vi "Write TaskConfig.vi"(8 "error in (no error)":errorcluster, 10 "TaskConfig":T1={"Drive"=enum."NI_DAQmx", "TaskType"=enum."AI", "PhysicalChannels"="", "SampleRateConfiguration"={"SampleRate"=0.0, "SamplesPerChannel"=0, "SamplesPerRead"=0, "SampleMode"=10123, "Clock Source"="OnboardClock"}, "ChannelConfig"={}, "Enable"=FALSE, "Original"=FALSE} {"SampleRateConfiguration"."SampleMode" items=["Finite Samples"=10178, "Continuous Samples"=10123, "Hardware Timed Single Point"=12522]}, 11 "Angular_Task in":refnum<class "Angular_Task.lvclass">) -> (0 "error out":errorcluster, 3 "Angular_Task out":refnum<class "Angular_Task.lvclass">)   [LabVIEW 2025, in "Angular_Task.lvlib" / "Angular_Task.lvclass"]
uses:
  Angular_Task.lvclass
  DAQ_Module/DAQ_Module/DAQ_Module/DAQ_Task_Config.ctl
  DAQ_Module/DAQ_Module/DAQ_Module/DAQ_HW_Type.ctl
  DAQ_Module/DAQ_Module/DAQ_Module/DAQ_Task_Type.ctl
  DAQ_Module/DAQ_Module/DAQ_Module/DAQ_SampleRateConfig.ctl
  DAQ_Module/DAQ_Module/DAQ_Module/DAQ_Angular_Task_Config.ctl
  e3aac5b7-c646-4fcd-a3ef-a0d2258a22a5.vi
  <vilib>/JDP Science/JSONtext/JSON text to Variant.vi
  Waveform_Task/Waveform_Task/Waveform_Task.lvclass
  <vilib>/JDP Science/JSONtext/LVClass Serializer/JSONtext LVClass Serializer.lvclass
  DAQ_Module/DAQ_Module/DAQ_Module/DAQ_Module.lvclass
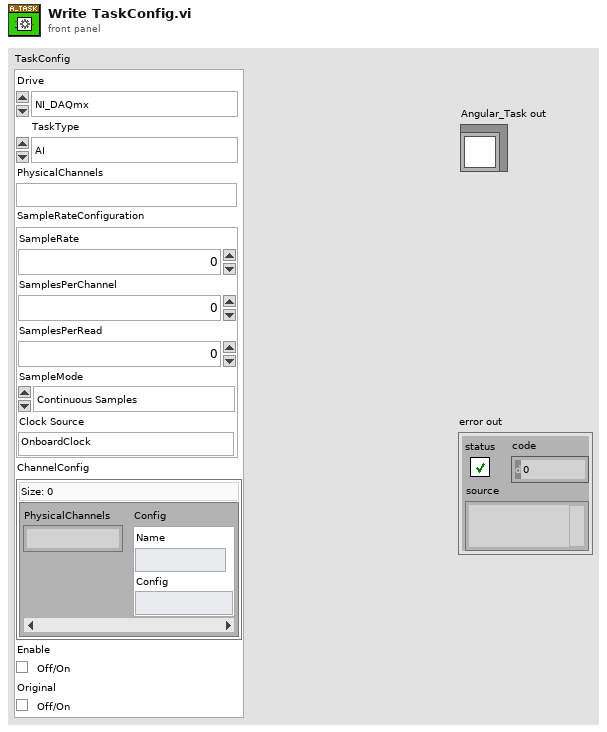
[diagram p1: front panel]
types:
  T1 = typedef "DAQ_Module.lvlib/DAQ_Module.lvclass/DAQ_Task_Config.ctl" = cluster{"Drive":T2, "TaskType":T3, "PhysicalChannels":string, "SampleRateConfiguration":T4, "ChannelConfig":map{string, cluster{"Name":string, "Config":string}}, "Enable":bool, "Original":bool}
  T2 = typedef "DAQ_Module.lvlib/DAQ_Module.lvclass/DAQ_HW_Type.ctl" = enum16{"NI_DAQmx", "Simulated_DAQ"}
  T3 = typedef "DAQ_Module.lvlib/DAQ_Module.lvclass/DAQ_Task_Type.ctl" = enum16{"AI", "Linear", "Angular", "AO"}
  T4 = typedef "DAQ_Module.lvlib/DAQ_Module.lvclass/DAQ_SampleRateConfig.ctl" = cluster{"SampleRate":dbl, "SamplesPerChannel":u32, "SamplesPerRead":i32, "SampleMode":i32, "Clock Source":string}
  T5 = typedef "DAQ_Module.lvlib/DAQ_Module.lvclass/DAQ_Angular_Task_Config.ctl" = cluster{"decoding type":i32, "units":i32, "pulses per revolution":u32, "initial angle":dbl, "z index enable":bool, "z index value":dbl, "z index phase":i32, "CI_Encoder_A_InputTerm":string, "CI_Encoder_B_InputTerm":string, "CI_Encoder_Z_InputTerm":string}
  T6 = map{string, cluster{"ChannelName":string, "AngularConfig":T5}}
  T7 = map{string, cluster{"Name":string, "Config":string}}
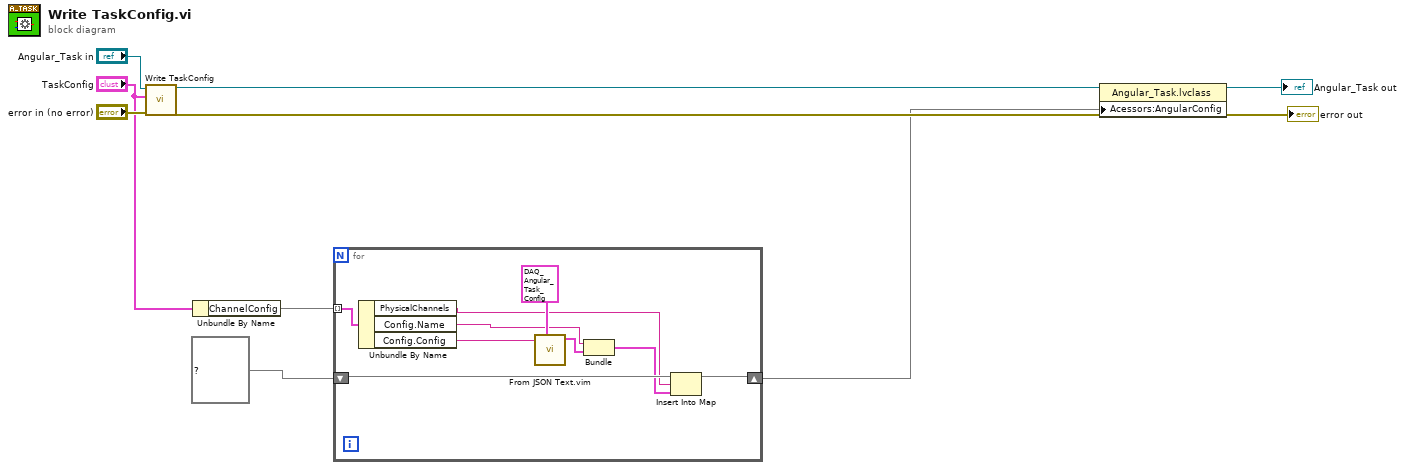
[diagram p0: block diagram]
diagram:
  n1 = call-parent "Write TaskConfig.vi"("error in (no error)"="error in (no error)", "TaskConfig"="TaskConfig", "Task_Abstr in"="Angular_Task in") -> ("error out"=→"error out":errorcluster, "Task_Abstr out"=w8:refnum<class "Angular_Task.lvclass">)  [unwired: 7 in]
  n2 = Unbundle By Name("TaskConfig") -> ("ChannelConfig"=w3:T7)
  n3 = for {
    tunnel: w3 -> [w16] mode=indexing
    shift-right: [w17] -> w1
    shift-left: T6 {} ("map") -> [w18]
    n4 = Unbundle By Name(w16) -> ("PhysicalChannels"=w10:string, "Config.Name"=w12:string, "Config.Config"=w15:string)
    n5 = call "From JSON Text.vim"("Data Type and Default Value"=T5 {"decoding type"=10092, "units"=10146, "pulses per revolution"=24, "initial angle"=0.0, "z index enable"=FALSE, "z index value"=0.0, "z index phase"=10040, "CI_Encoder_A_InputTerm"="", "CI_Encoder_B_InputTerm"="", "CI_Encoder_Z_InputTerm"=""} ("AngularConfig"), "JSON"=w15) -> ("Data out"=w13:T5)  [unwired: 8 in, 1 out]
    n6 = Bundle("Name"=w12, "Data out"=w13) -> (w11:cluster{"Name":string, "Data out":T5})  [unwired: 1 in]
    n7 = Insert Into Map(map in=w18, key=w10, value=w11) -> (map out=w17:T6)  [unwired: 2 out]
  }
  n8 = property class="Angular_Task.lvclass"(reference=w8, "Acessors:AngularConfig"=w1) -> (reference out=→"Angular_Task out":refnum<class "Angular_Task.lvclass">)  [unwired: 1 in, 1 out]
